vi "read_check_input.vi"(8 "error in (no error)":errorcluster, 11 "IncrementalPCA in":refnum<class "IncrementalPCA.lvclass">) -> (0 "error out":errorcluster, 2 "check_input":bool=TRUE, 3 "IncrementalPCA out":refnum<class "IncrementalPCA.lvclass">)   [LabVIEW 2020, in "IncrementalPCA.lvclass"]
uses:
  IncrementalPCA.lvclass
  IncrementalPCA.lvclass/IncrementalPCA.ctl
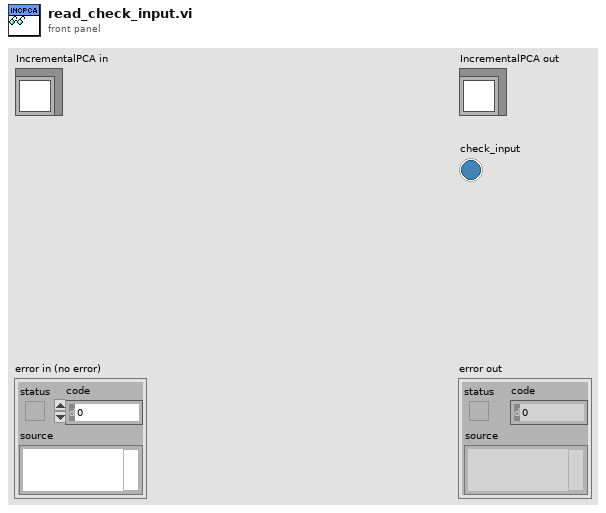
[diagram p1: front panel]
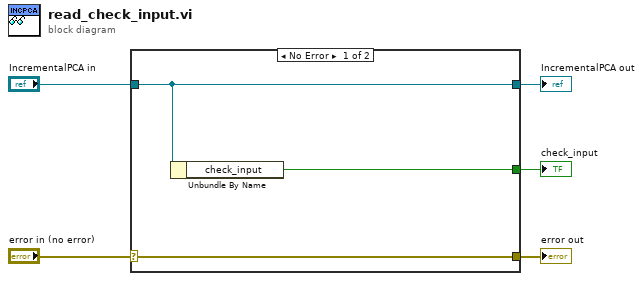
[diagram p0: block diagram]
diagram:
  n1 = case shown="No Error" "error in (no error)" {
    selector: "error in (no error)" -> [w8 w9]
    tunnel: [w8 w9] -> w4
    tunnel: [w7 w10] -> w2
    tunnel: "IncrementalPCA in" -> [w7 w10]
    tunnel: [w6 _] -> w1
    frame No Error {
      n2 = Unbundle By Name(w7) -> ("check_input"=w6:bool)
    }
    frame Error {
    }
  }
  "error out" <- w4
  "IncrementalPCA out" <- w2
  "check_input" <- w1
